vi "wiltron simple.vi"(10 "set f (MHz)":dbl=80.0 format="%#_13g", 11 "set P (dbm)":dbl=80.0 format="%#_13g") -> ()   [LabVIEW 2020]
panel:
  out "read buffer 2":string
  out "read buffer":string
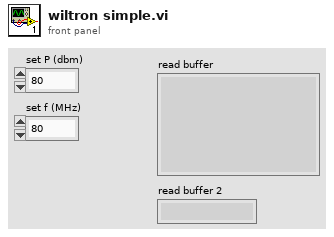
[diagram p1: front panel]
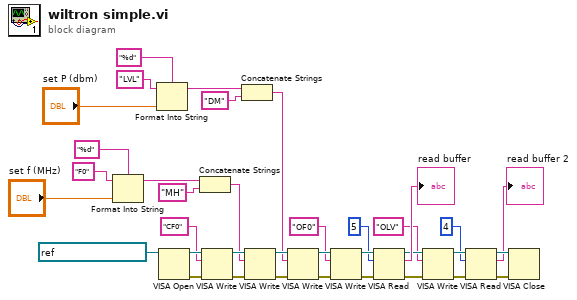
[diagram p0: block diagram]
diagram:
  n1 = Format Into String(format string="%d", initial string="F0", "set f (MHz)") -> (resulting string=w9:string)  [unwired: 1 in, 1 out]
  n2 = Format Into String(format string="%d", initial string="LVL", "set P (dbm)") -> (resulting string=w3:string)  [unwired: 1 in, 1 out]
  n3 = VISA Open(VISA resource name=refnum<visa-resource-name> "GPIB0::5::INSTR") -> (VISA resource name=w33:refnum<visa-resource-name>, error out=w35:errorcluster)  [unwired: 4 in]
  n4 = Concatenate Strings(w9, "MH" ("string")) -> (w7:string)
  n5 = VISA Write(VISA resource name=w33, write buffer="CF0", error in (no error)=w35) -> (VISA resource name out=w32:refnum<visa-resource-name>, error out=w34:errorcluster)  [unwired: 1 out]
  n6 = Concatenate Strings(w3, "DM" ("string")) -> (w1:string)
  n7 = VISA Write(VISA resource name=w32, write buffer=w7, error in (no error)=w34) -> (VISA resource name out=w30:refnum<visa-resource-name>, error out=w29:errorcluster)  [unwired: 1 out]
  n8 = VISA Write(VISA resource name=w30, write buffer=w1, error in (no error)=w29) -> (VISA resource name out=w27:refnum<visa-resource-name>, error out=w28:errorcluster)  [unwired: 1 out]
  n9 = VISA Write(VISA resource name=w27, write buffer="OF0", error in (no error)=w28) -> (VISA resource name out=w26:refnum<visa-resource-name>, error out=w25:errorcluster)  [unwired: 1 out]
  n10 = VISA Read(VISA resource name=w26, byte count=u32 5, error in (no error)=w25) -> (VISA resource name out=w18:refnum<visa-resource-name>, read buffer=→"read buffer":string, error out=w17:errorcluster)  [unwired: 1 out]
  n11 = VISA Write(VISA resource name=w18, write buffer="OLV", error in (no error)=w17) -> (VISA resource name out=w21:refnum<visa-resource-name>, error out=w20:errorcluster)  [unwired: 1 out]
  n12 = VISA Read(VISA resource name=w21, byte count=u32 4, error in (no error)=w20) -> (VISA resource name out=w15:refnum<visa-resource-name>, read buffer=→"read buffer 2":string, error out=w16:errorcluster)  [unwired: 1 out]
  n13 = VISA Close(VISA resource name=w15, error in (no error)=w16) -> ()  [unwired: 1 out]
